vi "检查账户.vi"(11 "密码":string) -> (1 "账户存在？":bool, 3 "账户信息":T1)   [LabVIEW 2018]
uses:
  <vilib>/Utility/file.llb/Read Delimited Spreadsheet (string).vi
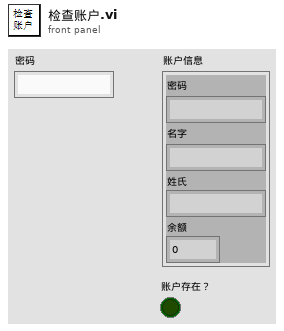
[diagram p1: front panel]
types:
  T1 = typedef "账户信息.ctl" = cluster{"密码":string, "名字":string, "姓氏":string, "余额":dbl}
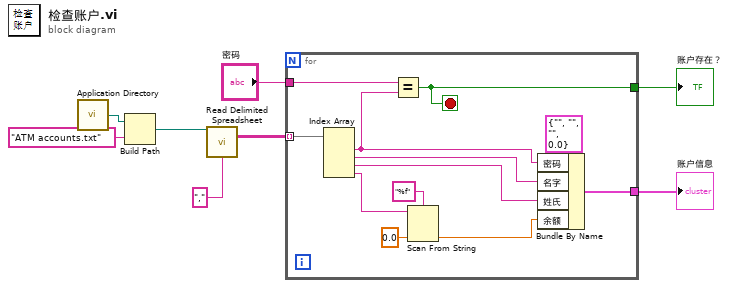
[diagram p0: block diagram]
diagram:
  n1 = call <vilib>:"Application Directory.vi"() -> ("Application Directory"=w8:path)
  n2 = Build Path(base path=w8, name or relative path="ATM accounts.txt" ("名称或相对路径")) -> (appended path=w6:path)
  n3 = call-poly <vilib>:"Read Delimited Spreadsheet.vi"("file path (dialog if empty)"=w6, "delimiter (\\t)"="," ("delimiter (\\t)")) -> ("all rows"=w4:string[][])  [unwired: 8 in, 5 out]
  n4 = for {
    tunnel: w4 -> [w20] mode=indexing
    tunnel: "密码" -> [w19]
    tunnel: [w17] -> w2
    tunnel: [w16] -> w1
    stop <- w16 stop-if-true
    n5 = Index Array(array=w20) -> (element #1=w15:string, element #2=w14:string, element #3=w13:string, element #4=w12:string)  [unwired: 4 in]
    n6 = Equal?(x=w19, y=w15) -> (x = y?=w16:bool)
    n7 = Scan From String(format string="%f" ("格式字符串"), input string=w12, default 1=0.0 ("默认值 1")) -> (output 1=w10:dbl)  [unwired: 2 in, 3 out]
    n8 = Bundle By Name(cluster=T1 {"密码"="", "名字"="", "姓氏"="", "余额"=0.0} ("账户信息"), "密码"=w15, "名字"=w14, "姓氏"=w13, "余额"=w10) -> (w17:T1)
  }
  "账户存在？" <- w1
  "账户信息" <- w2
